vi "Plot Electrical Data.vi"(0 "Plot Refnums":T1, 5 "Plot List":T3(tab), 7 "Electrical Measurement":T2, 9 "Measurement Mode":enum16{"Sweeping Mode", "Sampling Mode"}(ring), 11 "error in (no error)":errorcluster, 12 "Update Labels?":bool=TRUE, 13 "Update Pane?":bool) -> (4 "Voltage Plot Array":cluster{"Sequence":dbl[], "Data":dbl[]}[](array[cluster]), 6 "Current Plot Array":cluster{"Sequence":dbl[], "Data":dbl[]}[](array[cluster]), 8 "Current Voltage Array":cluster{"Voltage":dbl[], "Current":dbl[]}[](array[cluster]), 10 "Differential Resistance Array":cluster{"Voltage":dbl[], "Resistance":dbl[]}[](array[cluster]), 15 "error out":errorcluster)   [LabVIEW 2014]
uses:
  Hardware Control/Parameter Analyzer/Electrical Data.ctl
  Electrical Data Plot Refnums.ctl
panel:
  out "Current Plot 2":cluster{"Time":dbl[], "SMU4":dbl[]}[](graph)=[{"Time"=[0.0, 0.30000000000000004, 0.6000000000000001, 0.9, 1.2000000000000002, 1.5, 1.8, 2.1, 2.4000000000000004, 2.7, 3.0, 3.3000000000000003, 3.6, 3.9000000000000004, 4.2, 4.5, 4.800000000000001, 5.1000000000000005, 5.4, 5.7, 6.0, 6.300000000000001, 6.6000000000000005, 6.9, 7.2, 7.5, 7.800000000000001, 8.1, 8.4, 8.700000000000001, 9.0, 9.3, 9.600000000000001, 9.9, 10.200000000000001, 10.5, 10.8, 11.100000000000001, 11.4, 11.700000000000001, 12.0, 12.3, 12.600000000000001, 12.9, 13.200000000000001, 13.5, 13.8, 14.100000000000001, 14.4, 14.700000000000001, 15.0, 15.3, 15.600000000000001, 15.9, 16.2, 16.5, 16.8, 17.1, 17.400000000000002, 17.7], "SMU4"=[9.99995e-06, 9.99995e-06, 9.99995e-06, 9.99997e-06, 9.99997e-06, 9.99997e-06, 9.99997e-06, 9.999980000000001e-06, 9.99997e-06, 9.999980000000001e-06, 9.99997e-06, 9.999980000000001e-06, 9.99997e-06, 9.99997e-06, 9.99997e-06, 9.99996e-06, 9.99996e-06, 9.99996e-06, 9.99996e-06, 9.99997e-06, 9.99997e-06, 9.999980000000001e-06, 9.99997e-06, 9.99997e-06, 9.99997e-06, 9.99997e-06, 9.99997e-06, 9.999980000000001e-06, 9.999980000000001e-06, 9.99996e-06, 9.99997e-06, 9.99996e-06, 9.99997e-06, 9.99997e-06, 9.99997e-06, 9.99997e-06, 9.999980000000001e-06, 9.99997e-06, 9.999980000000001e-06, 9.999980000000001e-06, 9.99997e-06, 9.99997e-06, 9.99997e-06, 9.99996e-06, 9.99996e-06, 9.99997e-06, 9.99997e-06, 9.99996e-06, 9.99996e-06, 9.99997e-06, 9.99997e-06, 9.99997e-06, 9.99997e-06, 9.99997e-06, 9.99996e-06, 9.99997e-06, 9.99997e-06, 9.99997e-06, 9.99997e-06, 9.99996e-06]}, {"Time"=[0.0, 0.30000000000000004, 0.6000000000000001, 0.9, 1.2000000000000002, 1.5, 1.8, 2.1, 2.4000000000000004, 2.7, 3.0, 3.3000000000000003, 3.6, 3.9000000000000004, 4.2, 4.5, 4.800000000000001, 5.1000000000000005, 5.4, 5.7, 6.0, 6.300000000000001, 6.6000000000000005, 6.9, 7.2, 7.5, 7.800000000000001, 8.1, 8.4, 8.700000000000001, 9.0, 9.3, 9.600000000000001, 9.9, 10.200000000000001, 10.5, 10.8, 11.100000000000001, 11.4, 11.700000000000001, 12.0, 12.3, 12.600000000000001, 12.9, 13.200000000000001, 13.5, 13.8, 14.100000000000001, 14.4, 14.700000000000001, 15.0, 15.3, 15.600000000000001, 15.9, 16.2, 16.5, 16.8, 17.1, 17.400000000000002, 17.7], "SMU4"=[-1.00004e-05, -1.000039e-05, -1.000039e-05, -1.0000409999999999e-05, -1.000039e-05, -1.000039e-05, -1.00004e-05, -1.000043e-05, -1.000042e-05, -1.0000409999999999e-05, -1.000039e-05, -1.000039e-05, -1.0000409999999999e-05, -1.00004e-05, -1.000038e-05, -1.000038e-05, -1.000039e-05, -1.000037e-05, -1.000038e-05, -1.000039e-05, -1.000039e-05, -1.000039e-05, -1.000039e-05, -1.000039e-05, -1.00004e-05, -1.000037e-05, -1.000038e-05, -1.000039e-05, -1.00004e-05, -1.00004e-05, -1.00004e-05, -1.000037e-05, -1.000037e-05, -1.000037e-05, -1.000036e-05, -1.000039e-05, -1.000038e-05, -1.000037e-05, -1.000036e-05, -1.000037e-05, -1.000038e-05, -1.000037e-05, -1.000038e-05, -1.000036e-05, -1.000037e-05, -1.000037e-05, -1.000037e-05, -1.000039e-05, -1.000038e-05, -1.000036e-05, -1.000037e-05, -1.000039e-05, -1.000036e-05, -1.000037e-05, -1.000038e-05, -1.00004e-05, -1.0000409999999999e-05, -1.000038e-05, -1.000038e-05, -1.00004e-05]}]
  out "Voltage Plot 2":cluster{"Time":dbl[], "SMU4":dbl[]}[](graph)=[{"Time"=[0.0, 0.30000000000000004, 0.6000000000000001, 0.9, 1.2000000000000002, 1.5, 1.8, 2.1, 2.4000000000000004, 2.7, 3.0, 3.3000000000000003, 3.6, 3.9000000000000004, 4.2, 4.5, 4.800000000000001, 5.1000000000000005, 5.4, 5.7, 6.0, 6.300000000000001, 6.6000000000000005, 6.9, 7.2, 7.5, 7.800000000000001, 8.1, 8.4, 8.700000000000001, 9.0, 9.3, 9.600000000000001, 9.9, 10.200000000000001, 10.5, 10.8, 11.100000000000001, 11.4, 11.700000000000001, 12.0, 12.3, 12.600000000000001, 12.9, 13.200000000000001, 13.5, 13.8, 14.100000000000001, 14.4, 14.700000000000001, 15.0, 15.3, 15.600000000000001, 15.9, 16.2, 16.5, 16.8, 17.1, 17.400000000000002, 17.7], "SMU4"=[9.99995e-06, 9.99995e-06, 9.99995e-06, 9.99997e-06, 9.99997e-06, 9.99997e-06, 9.99997e-06, 9.999980000000001e-06, 9.99997e-06, 9.999980000000001e-06, 9.99997e-06, 9.999980000000001e-06, 9.99997e-06, 9.99997e-06, 9.99997e-06, 9.99996e-06, 9.99996e-06, 9.99996e-06, 9.99996e-06, 9.99997e-06, 9.99997e-06, 9.999980000000001e-06, 9.99997e-06, 9.99997e-06, 9.99997e-06, 9.99997e-06, 9.99997e-06, 9.999980000000001e-06, 9.999980000000001e-06, 9.99996e-06, 9.99997e-06, 9.99996e-06, 9.99997e-06, 9.99997e-06, 9.99997e-06, 9.99997e-06, 9.999980000000001e-06, 9.99997e-06, 9.999980000000001e-06, 9.999980000000001e-06, 9.99997e-06, 9.99997e-06, 9.99997e-06, 9.99996e-06, 9.99996e-06, 9.99997e-06, 9.99997e-06, 9.99996e-06, 9.99996e-06, 9.99997e-06, 9.99997e-06, 9.99997e-06, 9.99997e-06, 9.99997e-06, 9.99996e-06, 9.99997e-06, 9.99997e-06, 9.99997e-06, 9.99997e-06, 9.99996e-06]}, {"Time"=[0.0, 0.30000000000000004, 0.6000000000000001, 0.9, 1.2000000000000002, 1.5, 1.8, 2.1, 2.4000000000000004, 2.7, 3.0, 3.3000000000000003, 3.6, 3.9000000000000004, 4.2, 4.5, 4.800000000000001, 5.1000000000000005, 5.4, 5.7, 6.0, 6.300000000000001, 6.6000000000000005, 6.9, 7.2, 7.5, 7.800000000000001, 8.1, 8.4, 8.700000000000001, 9.0, 9.3, 9.600000000000001, 9.9, 10.200000000000001, 10.5, 10.8, 11.100000000000001, 11.4, 11.700000000000001, 12.0, 12.3, 12.600000000000001, 12.9, 13.200000000000001, 13.5, 13.8, 14.100000000000001, 14.4, 14.700000000000001, 15.0, 15.3, 15.600000000000001, 15.9, 16.2, 16.5, 16.8, 17.1, 17.400000000000002, 17.7], "SMU4"=[-1.00004e-05, -1.000039e-05, -1.000039e-05, -1.0000409999999999e-05, -1.000039e-05, -1.000039e-05, -1.00004e-05, -1.000043e-05, -1.000042e-05, -1.0000409999999999e-05, -1.000039e-05, -1.000039e-05, -1.0000409999999999e-05, -1.00004e-05, -1.000038e-05, -1.000038e-05, -1.000039e-05, -1.000037e-05, -1.000038e-05, -1.000039e-05, -1.000039e-05, -1.000039e-05, -1.000039e-05, -1.000039e-05, -1.00004e-05, -1.000037e-05, -1.000038e-05, -1.000039e-05, -1.00004e-05, -1.00004e-05, -1.00004e-05, -1.000037e-05, -1.000037e-05, -1.000037e-05, -1.000036e-05, -1.000039e-05, -1.000038e-05, -1.000037e-05, -1.000036e-05, -1.000037e-05, -1.000038e-05, -1.000037e-05, -1.000038e-05, -1.000036e-05, -1.000037e-05, -1.000037e-05, -1.000037e-05, -1.000039e-05, -1.000038e-05, -1.000036e-05, -1.000037e-05, -1.000039e-05, -1.000036e-05, -1.000037e-05, -1.000038e-05, -1.00004e-05, -1.0000409999999999e-05, -1.000038e-05, -1.000038e-05, -1.00004e-05]}]
  out "Differential Resistance":cluster{"V3":dbl[], "I1":dbl[]}[](graph)
  out "Current Voltage Characteristic":cluster{"V3":dbl[], "I1":dbl[]}[](graph)
  # "LICENSED MATERIALS – PROPERTY OF IBM\nCopyright IBM Corp. 2016,\nALL RIGHTS RESERVED"
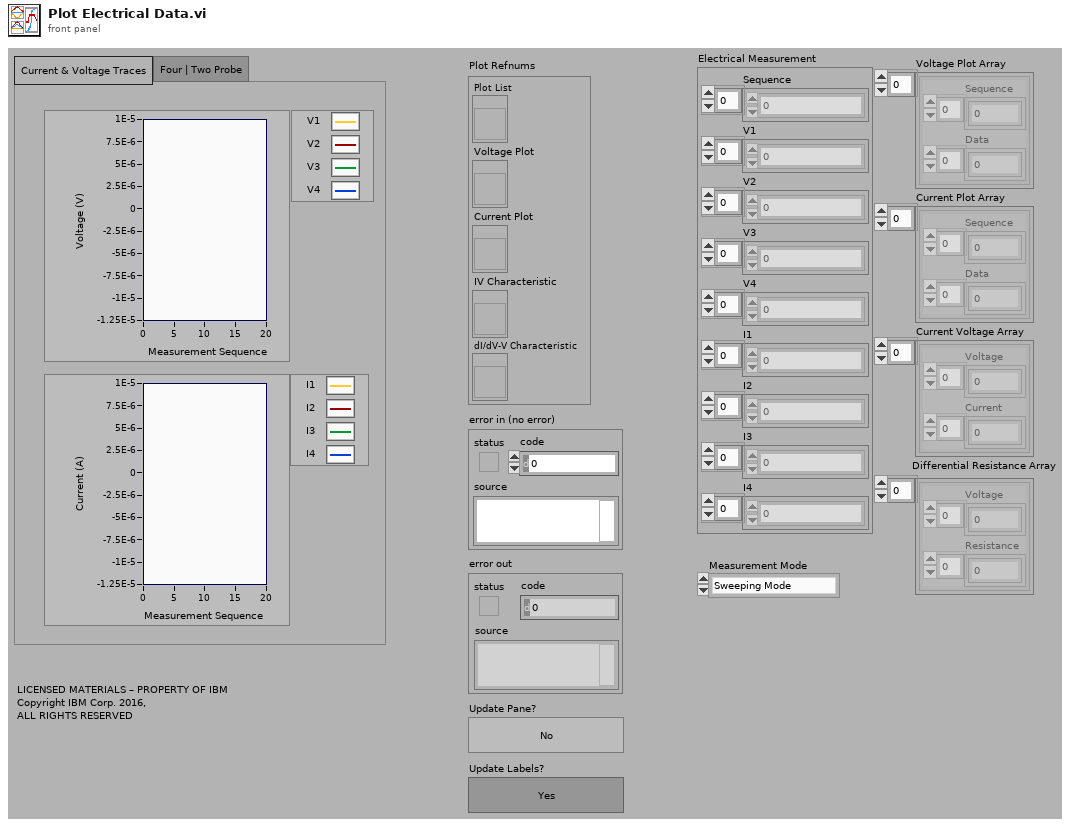
[diagram p1: front panel]
types:
  T1 = typedef "Electrical Data Plot Refnums.ctl" = cluster{"Plot List":refnum<vi>, "Voltage Plot":refnum<vi>, "Current Plot":refnum<vi>, "IV Characteristic":refnum<vi>, "dI/dV-V Characteristic":refnum<vi>}
  T2 = typedef "Electrical Data.ctl" = cluster{"Sequence":dbl[], "V1":dbl[], "V2":dbl[], "V3":dbl[], "V4":dbl[], "I1":dbl[], "I2":dbl[], "I3":dbl[], "I4":dbl[]}
  T3 = enum32{"Current & Voltage Traces", "Four | Two Probe"}
  T4 = cluster{"Voltage":dbl[], "4-Point Resistance":dbl[]}[]
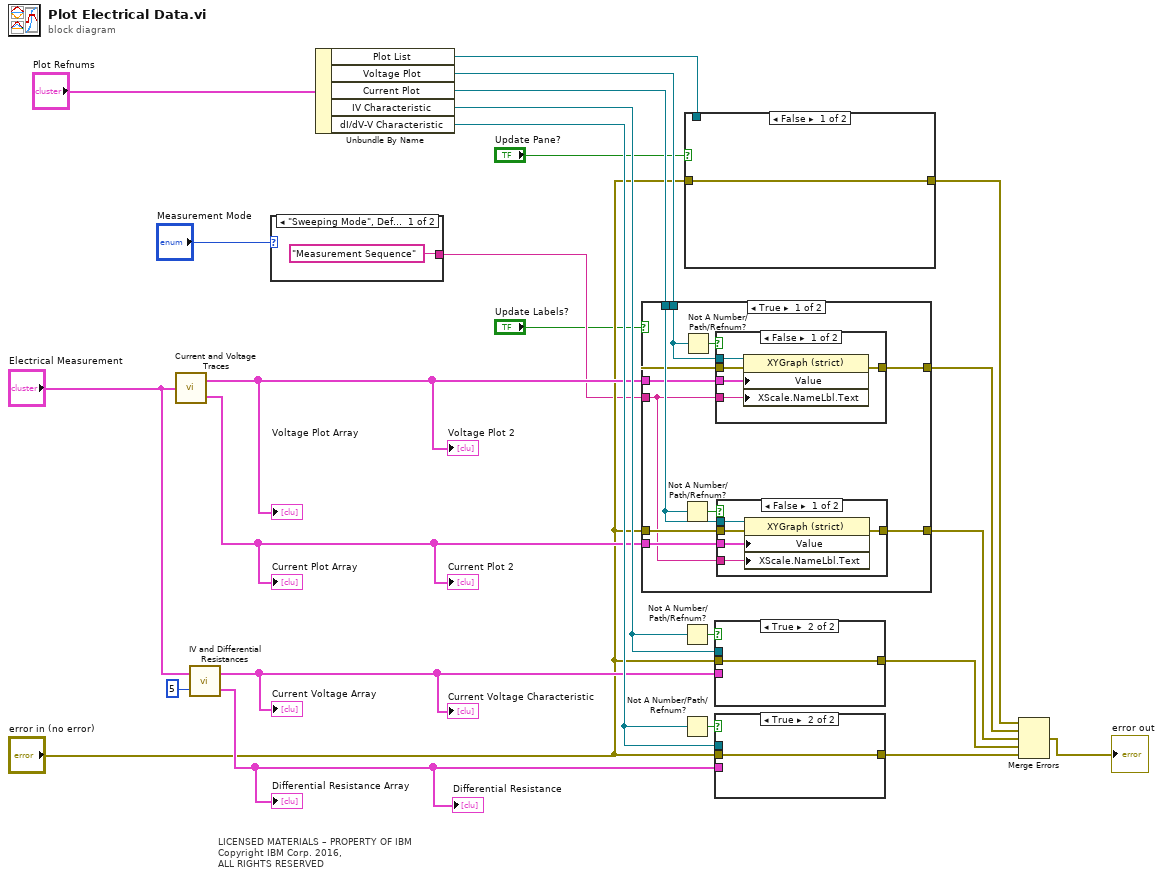
[diagram p0: block diagram]
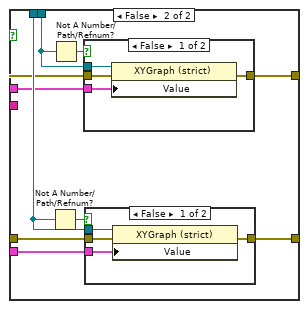
[diagram p4: hidden frame]
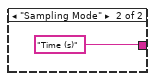
[diagram p7: hidden frame]
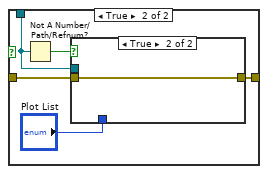
[diagram p8: hidden frame]
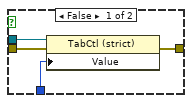
[diagram p9: hidden frame]
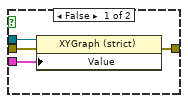
[diagram p10: hidden frame]
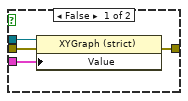
[diagram p11: hidden frame]
diagram:
  # "LICENSED MATERIALS – PROPERTY OF IBM\nCopyright IBM Corp. 2016,\nALL RIGHTS RESERVED"
  n1 = call "Current and Voltage Traces.vi"("Measurement"="Electrical Measurement") -> ("Current Plot"=w11:cluster{"Sequence":dbl[], "Data":dbl[]}[], "Voltage Plot"=w16:cluster{"Sequence":dbl[], "Data":dbl[]}[])  [unwired: 2 out]
  "Voltage Plot 2" <- w16
  "Current Plot 2" <- w11
  "Voltage Plot Array" <- w16
  "Current Plot Array" <- w11
  n2 = call "IV and Differential Resistances.vi"("Derivative Interval"=5, "Electrical Measurement"="Electrical Measurement") -> ("Differential Resistances"=w9:T4, "Current Voltage-Characteristics"=w10:cluster{"Voltage":dbl[], "Current":dbl[]}[])
  "Current Voltage Characteristic" <- w10
  "Differential Resistance" <- w9
  "Current Voltage Array" <- w10
  "Differential Resistance Array" <- w9
  n3 = case shown="\"Sweeping Mode\", Default" "Measurement Mode" {
    tunnel: ["Measurement Sequence" "Time (s)"] -> w3
    frame "Sweeping Mode", Default {
    }
    frame "Sampling Mode" {
    }
  }
  n4 = Unbundle By Name("Plot Refnums") -> ("Plot List"=w7:refnum<vi>, "Voltage Plot"=w17:refnum<vi>, "Current Plot"=w18:refnum<vi>, "IV Characteristic"=w19:refnum<vi>, "dI/dV-V Characteristic"=w20:refnum<vi>)
  n5 = case shown="True" "Update Labels?" {
    tunnel: w18 -> [w36 w57]
    tunnel: w17 -> [w35 w56]
    tunnel: w16 -> [w34 w55]
    tunnel: [w33 w54] -> w13
    tunnel: [w32 w53] -> w12
    tunnel: w11 -> [w31 w52]
    tunnel: "error in (no error)" -> [w30 w51]
    tunnel: w3 -> [w29 _]
    frame True {
      n6 = Not A Number/Path/Refnum?(number/path/refnum=w36) -> (NaN/Path/Refnum?=w37:bool)
      n7 = Not A Number/Path/Refnum?(number/path/refnum=w35) -> (NaN/Path/Refnum?=w28:bool)
      n8 = case shown="False" w28 {
        tunnel: w35 -> [w42 _]
        tunnel: w34 -> [w41 _]
        tunnel: w30 -> [w40 w43]
        tunnel: [w39 w43] -> w32
        tunnel: w29 -> [w38 _]
        frame False {
          n9 = property class="XYGraph (strict)"(reference=w42, error in=w40, "Value"=w41, "XScale.NameLbl.Text"=w38) -> (error out=w39:errorcluster)  [unwired: 1 out]
        }
        frame True {
        }
      }
      n10 = case shown="False" w37 {
        tunnel: w36 -> [w48 _]
        tunnel: w31 -> [w47 _]
        tunnel: w30 -> [w46 w49]
        tunnel: [w45 w49] -> w33
        tunnel: w29 -> [w44 _]
        frame False {
          n11 = property class="XYGraph (strict)"(reference=w48, error in=w46, "Value"=w47, "XScale.NameLbl.Text"=w44) -> (error out=w45:errorcluster)  [unwired: 1 out]
        }
        frame True {
        }
      }
    }
    frame False {
      n12 = Not A Number/Path/Refnum?(number/path/refnum=w57) -> (NaN/Path/Refnum?=w58:bool)
      n13 = Not A Number/Path/Refnum?(number/path/refnum=w56) -> (NaN/Path/Refnum?=w50:bool)
      n14 = case shown="False" w50 {
        tunnel: w56 -> [w62 _]
        tunnel: w55 -> [w61 _]
        tunnel: w51 -> [w60 w63]
        tunnel: [w59 w63] -> w53
        frame False {
          n15 = property class="XYGraph (strict)"(reference=w62, error in=w60, "Value"=w61) -> (error out=w59:errorcluster)  [unwired: 1 out]
        }
        frame True {
        }
      }
      n16 = case shown="False" w58 {
        tunnel: w57 -> [w67 _]
        tunnel: w52 -> [w66 _]
        tunnel: w51 -> [w65 w68]
        tunnel: [w64 w68] -> w54
        frame False {
          n17 = property class="XYGraph (strict)"(reference=w67, error in=w65, "Value"=w66) -> (error out=w64:errorcluster)  [unwired: 1 out]
        }
        frame True {
        }
      }
    }
  }
  n18 = Not A Number/Path/Refnum?(number/path/refnum=w19) -> (NaN/Path/Refnum?=w21:bool)
  n19 = Not A Number/Path/Refnum?(number/path/refnum=w20) -> (NaN/Path/Refnum?=w22:bool)
  n20 = case shown="False" "Update Pane?" {
    tunnel: "error in (no error)" -> [w69 w74]
    tunnel: w7 -> [_ w72]
    tunnel: [w69 w70] -> w5
    frame False {
    }
    frame True {
      n21 = Not A Number/Path/Refnum?(number/path/refnum=w72) -> (NaN/Path/Refnum?=w73:bool)
      n22 = case shown="True" w73 {
        tunnel: [w78 w79] -> w70
        tunnel: w74 -> [w77 w79]
        tunnel: w72 -> [w76 _]
        tunnel: "Plot List" -> [w75 _]
        frame False {
          n23 = property class="TabCtl (strict)"(reference=w76, error in=w77, "Value"=w75) -> (error out=w78:errorcluster)  [unwired: 1 out]
        }
        frame True {
        }
      }
    }
  }
  n24 = case shown="True" w21 {
    tunnel: w19 -> [w83 _]
    tunnel: w10 -> [w82 _]
    tunnel: "error in (no error)" -> [w81 w84]
    tunnel: [w80 w84] -> w14
    frame False {
      n25 = property class="XYGraph (strict)"(reference=w83, error in=w81, "Value"=w82) -> (error out=w80:errorcluster)  [unwired: 1 out]
    }
    frame True {
    }
  }
  n26 = case shown="True" w22 {
    tunnel: "error in (no error)" -> [w88 w89]
    tunnel: w20 -> [w87 _]
    tunnel: w9 -> [w86 _]
    tunnel: [w85 w89] -> w15
    frame False {
      n27 = property class="XYGraph (strict)"(reference=w87, error in=w88, "Value"=w86) -> (error out=w85:errorcluster)  [unwired: 1 out]
    }
    frame True {
    }
  }
  n28 = Merge Errors(w5, w12, w13, w14, w15) -> (→"error out":errorcluster)
